vi "生成报告.vi"(0 "打印?":bool, 2 "输出簇":T1) -> ()   [LabVIEW 2010]
uses:
  <vilib>/Utility/NIReport.llb/NI_report.lvclass
  <vilib>/Utility/NIReport.llb/Append Report Text (str wrap).vi
  <vilib>/addons/_office/word.llb/Word Easy Table (str).vi
  <vilib>/addons/_office/NI_ReportGenerationToolkit.lvlib
panel:
  in  "序号":i32
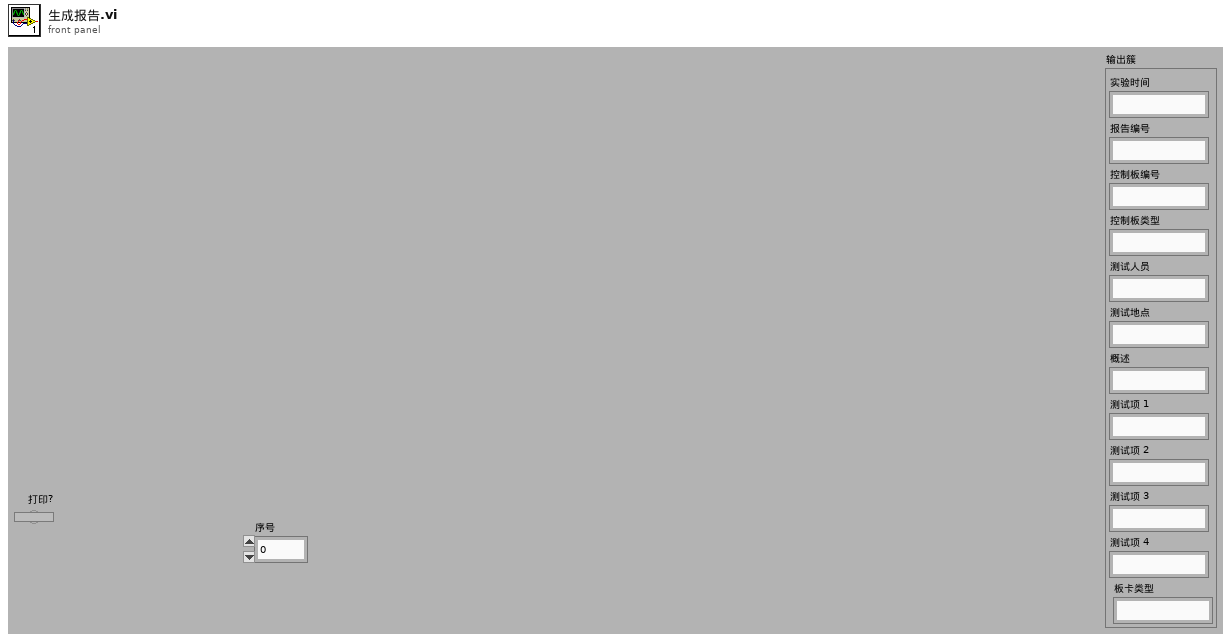
[diagram p1: front panel]
types:
  T1 = cluster{"实验时间":string, "报告编号":string, "控制板编号":string, "控制板类型":string, "测试人员":string, "测试地点":string, "概述":string, "测试项 1":string, "测试项 2":string, "测试项 3":string, "测试项 4":string, "板卡类型":string}
  T2 = cluster{"position (Excel)":cluster{"row":i32, "column":i32}, "name (Excel)":string, "bookmark (Word)":string}
  T3 = enum16{"maximized", "minimized", "normal", "no change"}
  T4 = enum16{"Standard Report", "HTML", "Word", "Excel"}
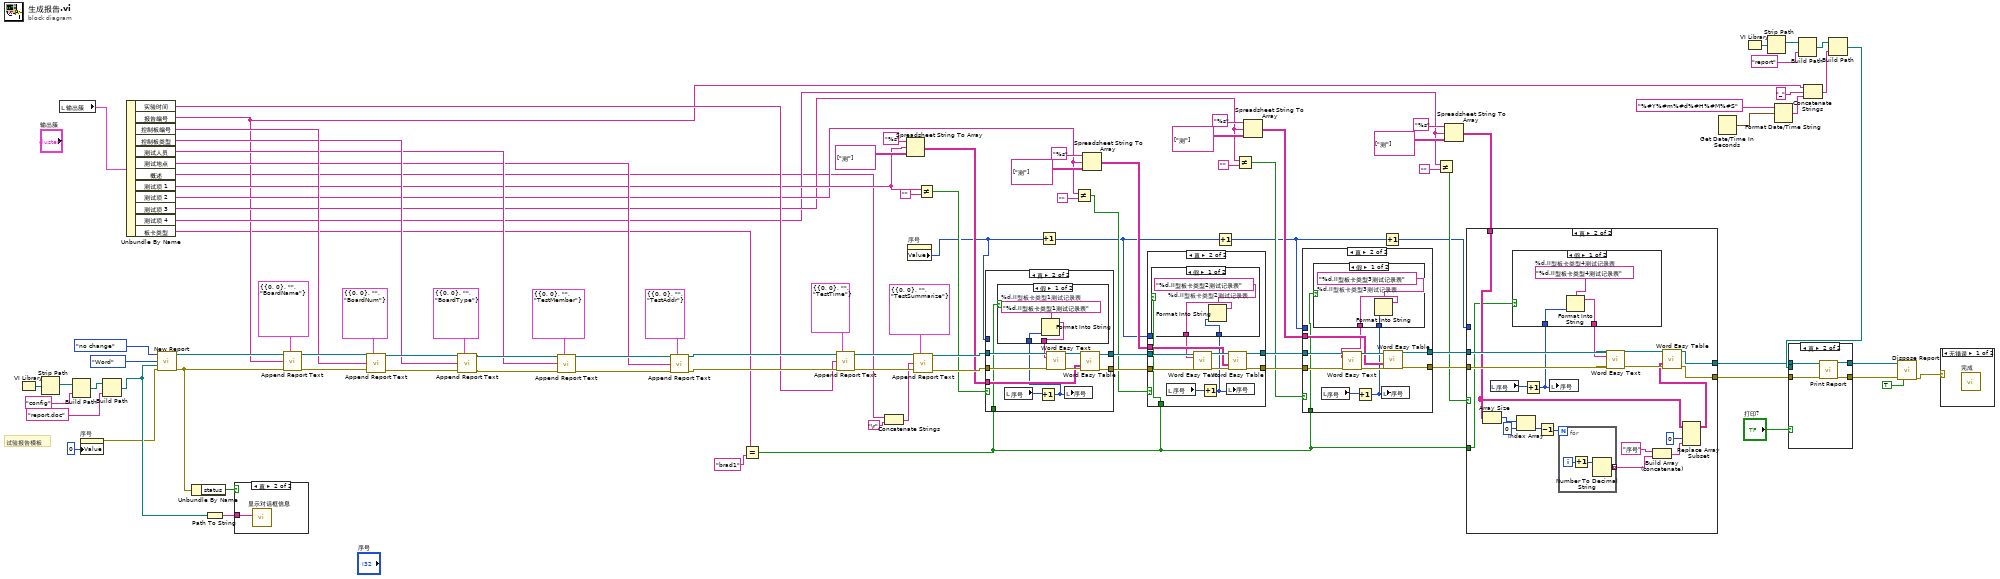
[diagram p0: block diagram]
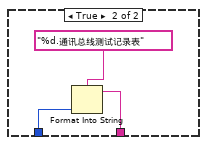
[diagram p3: hidden frame]
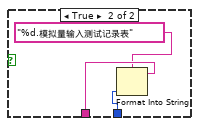
[diagram p5: hidden frame]
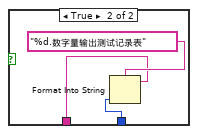
[diagram p7: hidden frame]
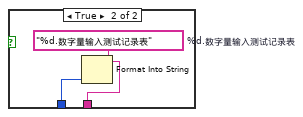
[diagram p9: hidden frame]
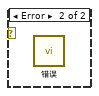
[diagram p10: hidden frame]
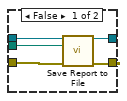
[diagram p11: hidden frame]
diagram:
  # "试验报告模板"
  n1 = VI Library() -> (path=w93:path)
  n2 = Strip Path(path=w93) -> (stripped path=w90:path)  [unwired: 1 out]
  n3 = local read "输出簇"() -> (w99:T1)
  n4 = Build Path(base path=w90, name or relative path="config") -> (appended path=w92:path)
  n5 = property on="序号" class="DigNum (严格)"("Value"=0 ("序号")) -> (error out=w44:errorcluster)  [unwired: 2 in, 1 out]
  n6 = Build Path(base path=w92, name or relative path="report.doc") -> (appended path=w96:path)
  n7 = Unbundle By Name(w99) -> ("实验时间"=w36:string, "报告编号"=w11:string, "控制板编号"=w40:string, "控制板类型"=w39:string, "测试人员"=w38:string, "测试地点"=w37:string, "概述"=w10:string, "测试项 1"=w31:string, "测试项 2"=w26:string, "测试项 3"=w20:string, "测试项 4"=w14:string, "板卡类型"=w2:string)
  n8 = call <vilib>:"New Report.vi"("window state (normal)"=T3."no change", "report type"=T4."Word", "template (empty)"=w96, "error in (no error)"=w44) -> ("report out"=w87:refnum<class "NI_report.lvclass">, "error out"=w86:errorcluster)  [unwired: 10 in]
  n9 = Unbundle By Name(w86) -> ("status"=w98:bool)
  n10 = Path To String(path=w96) -> (string=w97:string)
  n11 = case shown="真" w98 {
    tunnel: w97 -> [_ w100]
    frame False {
    }
    frame True {
      n12 = call "显示对话框信息"("Message"=w100) -> ()  [unwired: 9 in, 2 out]
    }
  }
  n13 = call-poly <vilib>:"Append Report Text.vi"("report in"=w87, "MS Office parameters"=T2 {"position (Excel)"={"row"=0, "column"=0}, "name (Excel)"="", "bookmark (Word)"="BoardName"}, "text"=w11, "error in (no error)"=w86) -> ("report out"=w72:refnum<class "NI_report.lvclass">, "error out"=w71:errorcluster)  [unwired: 8 in, 2 out]
  n14 = call-poly <vilib>:"Append Report Text.vi"("report in"=w72, "MS Office parameters"=T2 {"position (Excel)"={"row"=0, "column"=0}, "name (Excel)"="", "bookmark (Word)"="BoardNum"}, "text"=w40, "error in (no error)"=w71) -> ("report out"=w82:refnum<class "NI_report.lvclass">, "error out"=w81:errorcluster)  [unwired: 8 in, 2 out]
  n15 = call-poly <vilib>:"Append Report Text.vi"("report in"=w82, "MS Office parameters"=T2 {"position (Excel)"={"row"=0, "column"=0}, "name (Excel)"="", "bookmark (Word)"="BoardType"}, "text"=w39, "error in (no error)"=w81) -> ("report out"=w79:refnum<class "NI_report.lvclass">, "error out"=w78:errorcluster)  [unwired: 8 in, 2 out]
  n16 = call-poly <vilib>:"Append Report Text.vi"("report in"=w79, "MS Office parameters"=T2 {"position (Excel)"={"row"=0, "column"=0}, "name (Excel)"="", "bookmark (Word)"="TestMember"}, "text"=w38, "error in (no error)"=w78) -> ("report out"=w76:refnum<class "NI_report.lvclass">, "error out"=w75:errorcluster)  [unwired: 8 in, 2 out]
  n17 = call-poly <vilib>:"Append Report Text.vi"("report in"=w76, "MS Office parameters"=T2 {"position (Excel)"={"row"=0, "column"=0}, "name (Excel)"="", "bookmark (Word)"="TestAddr"}, "text"=w37, "error in (no error)"=w75) -> ("report out"=w74:refnum<class "NI_report.lvclass">, "error out"=w73:errorcluster)  [unwired: 8 in, 2 out]
  n18 = Equal?(x=w2, y="brad1") -> (x = y?=w1:bool)
  n19 = call-poly <vilib>:"Append Report Text.vi"("report in"=w74, "MS Office parameters"=T2 {"position (Excel)"={"row"=0, "column"=0}, "name (Excel)"="", "bookmark (Word)"="TestTime"}, "text"=w36, "error in (no error)"=w73) -> ("report out"=w49:refnum<class "NI_report.lvclass">, "error out"=w48:errorcluster)  [unwired: 8 in, 2 out]
  n20 = Concatenate Strings(w10, "\r") -> (w8:string)
  n21 = Spreadsheet String To Array(format string="%s" ("格式字符串"), spreadsheet string=w31, array type (2D Dbl)=string[][] [["测"]] ("数组类型(2D String)")) -> (array=w30:string[][])  [unwired: 1 in]
  n22 = property on="序号" class="DigNum (严格)"() -> ("Value"=w7:i32)  [unwired: 2 in, 2 out]
  n23 = call-poly <vilib>:"Append Report Text.vi"("report in"=w49, "MS Office parameters"=T2 {"position (Excel)"={"row"=0, "column"=0}, "name (Excel)"="", "bookmark (Word)"="TestSummarize"}, "text"=w8, "error in (no error)"=w48) -> ("report out"=w47:refnum<class "NI_report.lvclass">, "error out"=w46:errorcluster)  [unwired: 8 in, 2 out]
  n24 = Not Equal?(x=w31, y="") -> (x != y?=w34:bool)
  n25 = case shown="真" w34 {
    tunnel: [w102 w112] -> w56
    tunnel: [w101 w111] -> w54
    tunnel: w47 -> [w102 w109]
    tunnel: w46 -> [w101 w108]
    tunnel: w7 -> [_ _]
    tunnel: w30 -> [_ w107]
    tunnel: w1 -> [_ w105]
    frame False {
    }
    frame True {
      n26 = local read "序号"() -> (w104:i32)
      n27 = Increment(x=w104) -> (x+1=w103:i32)
      n28 = case shown="假" w105 {
        tunnel: [w115 w117] -> w106
        tunnel: w103 -> [w114 w119]
        frame False {
          w116 = "%d.II型板卡类型1测试记录表"  # %d.II型板卡类型1测试记录表
          n29 = Format Into String(format string=w116, w114) -> (resulting string=w115:string)  [unwired: 2 in, 1 out]
        }
        frame True {
          w118 = "%d.数字量输入测试记录表"  # %d.数字量输入测试记录表
          n30 = Format Into String(format string=w118, w119) -> (resulting string=w117:string)  [unwired: 2 in, 1 out]
        }
      }
      n31 = call <vilib>:"Word Easy Text.vi"("report in"=w109, "text"=w106, "error in (no error)"=w108) -> ("report out"=w113:refnum<class "NI_report.lvclass">, "error out"=w110:errorcluster)  [unwired: 10 in, 1 out]
      n32 = local write "序号"(w103) -> ()
      n33 = call-poly <vilib>:"Word Easy Table.vi"("report in"=w113, "data"=w107, "error in (no error)"=w110) -> ("report out"=w112:refnum<class "NI_report.lvclass">, "error out"=w111:errorcluster)  [unwired: 10 in, 1 out]
    }
  }
  n34 = Increment(x=w7) -> (x+1=w6:i32)
  n35 = Not Equal?(x=w26, y="") -> (x != y?=w25:bool)
  n36 = Spreadsheet String To Array(format string="%s" ("格式字符串"), spreadsheet string=w26, array type (2D Dbl)=string[][] [["测"]] ("数组类型(2D String)")) -> (array=w24:string[][])  [unwired: 1 in]
  n37 = case shown="真" w25 {
    tunnel: w56 -> [w121 w132]
    tunnel: [w121 w130] -> w55
    tunnel: w54 -> [w120 w129]
    tunnel: [w120 w127] -> w53
    tunnel: w6 -> [_ _]
    tunnel: w24 -> [_ w126]
    tunnel: w1 -> [_ w124]
    frame False {
    }
    frame True {
      n38 = local read "序号"() -> (w123:i32)
      n39 = Increment(x=w123) -> (x+1=w122:i32)
      n40 = case shown="假" w124 {
        tunnel: [w134 w136] -> w125
        tunnel: w122 -> [w135 w138]
        frame False {
          w133 = "%d.II型板卡类型2测试记录表"  # %d.II型板卡类型2测试记录表
          n41 = Format Into String(format string=w133, w135) -> (resulting string=w134:string)  [unwired: 2 in, 1 out]
        }
        frame True {
          n42 = Format Into String(format string="%d.数字量输出测试记录表", w138) -> (resulting string=w136:string)  [unwired: 2 in, 1 out]
        }
      }
      n43 = call <vilib>:"Word Easy Text.vi"("report in"=w132, "text"=w125, "error in (no error)"=w129) -> ("report out"=w131:refnum<class "NI_report.lvclass">, "error out"=w128:errorcluster)  [unwired: 10 in, 1 out]
      n44 = local write "序号"(w122) -> ()
      n45 = call-poly <vilib>:"Word Easy Table.vi"("report in"=w131, "data"=w126, "error in (no error)"=w128) -> ("report out"=w130:refnum<class "NI_report.lvclass">, "error out"=w127:errorcluster)  [unwired: 10 in, 1 out]
    }
  }
  n46 = Increment(x=w6) -> (x+1=w5:i32)
  n47 = Not Equal?(x=w20, y="") -> (x != y?=w19:bool)
  n48 = Spreadsheet String To Array(format string="%s" ("格式字符串"), spreadsheet string=w20, array type (2D Dbl)=string[][] [["测"]] ("数组类型(2D String)")) -> (array=w18:string[][])  [unwired: 1 in]
  n49 = case shown="真" w19 {
    tunnel: w55 -> [w140 w151]
    tunnel: w53 -> [w139 w149]
    tunnel: [w140 w147] -> w52
    tunnel: [w139 w146] -> w51
    tunnel: w5 -> [_ _]
    tunnel: w18 -> [_ w145]
    tunnel: w1 -> [_ w143]
    frame False {
    }
    frame True {
      n50 = local read "序号"() -> (w142:i32)
      n51 = Increment(x=w142) -> (x+1=w141:i32)
      n52 = case shown="假" w143 {
        tunnel: [w153 w156] -> w144
        tunnel: w141 -> [w154 w157]
        frame False {
          w152 = "%d.II型板卡类型3测试记录表"  # %d.II型板卡类型3测试记录表
          n53 = Format Into String(format string=w152, w154) -> (resulting string=w153:string)  [unwired: 2 in, 1 out]
        }
        frame True {
          n54 = Format Into String(format string="%d.模拟量输入测试记录表", w157) -> (resulting string=w156:string)  [unwired: 2 in, 1 out]
        }
      }
      n55 = call <vilib>:"Word Easy Text.vi"("report in"=w151, "text"=w144, "error in (no error)"=w149) -> ("report out"=w150:refnum<class "NI_report.lvclass">, "error out"=w148:errorcluster)  [unwired: 10 in, 1 out]
      n56 = local write "序号"(w141) -> ()
      n57 = call-poly <vilib>:"Word Easy Table.vi"("report in"=w150, "data"=w145, "error in (no error)"=w148) -> ("report out"=w147:refnum<class "NI_report.lvclass">, "error out"=w146:errorcluster)  [unwired: 10 in, 1 out]
    }
  }
  n58 = Increment(x=w5) -> (x+1=w4:i32)
  n59 = Not Equal?(x=w14, y="") -> (x != y?=w13:bool)
  n60 = Spreadsheet String To Array(format string="%s" ("格式字符串"), spreadsheet string=w14, array type (2D Dbl)=string[][] [["测"]] ("数组类型(2D String)")) -> (array=w12:string[][])  [unwired: 1 in]
  n61 = case shown="真" w13 {
    tunnel: [w159 w179] -> w58
    tunnel: [w158 w178] -> w57
    tunnel: w52 -> [w159 w177]
    tunnel: w51 -> [w158 w176]
    tunnel: w4 -> [_ _]
    tunnel: w12 -> [_ w164]
    tunnel: w1 -> [_ w162]
    frame False {
    }
    frame True {
      n62 = Array Size(array=w164) -> (size(s)=w165:i32[])
      n63 = local read "序号"() -> (w161:i32)
      n64 = Index Array(array=w165, index=0 ("索引")) -> (element=w168:i32)
      n65 = Increment(x=w161) -> (x+1=w160:i32)
      n66 = case shown="假" w162 {
        tunnel: [w182 w185] -> w173
        tunnel: w160 -> [w180 w183]
        frame False {
          w181 = "%d.II型板卡类型4测试记录表"  # %d.II型板卡类型4测试记录表
          n67 = Format Into String(format string=w181, w180) -> (resulting string=w182:string)  [unwired: 2 in, 1 out]
        }
        frame True {
          n68 = Format Into String(format string="%d.通讯总线测试记录表", w183) -> (resulting string=w185:string)  [unwired: 2 in, 1 out]
        }
      }
      n69 = Decrement(x=w168) -> (x-1=w169:i32)
      n70 = local write "序号"(w160) -> ()
      n71 = for {
        N: w169 -> [_]
        tunnel: [w186] -> w171 mode=indexing
        i -> [w188]
        n72 = Increment(x=w188) -> (x+1=w187:i32)
        n73 = Number To Decimal String(number=w187) -> (decimal integer string=w186:string)  [unwired: 1 in]
      }
      n74 = call <vilib>:"Word Easy Text.vi"("report in"=w177, "text"=w173, "error in (no error)"=w176) -> ("report out"=w175:refnum<class "NI_report.lvclass">, "error out"=w174:errorcluster)  [unwired: 10 in, 1 out]
      n75 = Build Array (concatenate)("序号", w171) -> (w172:string[])
      n76 = Replace Array Subset(array=w164, new element=w172, index (col)=0 ("索引 (行)")) -> (w163:string[][])  [unwired: 1 in]
      n77 = call-poly <vilib>:"Word Easy Table.vi"("report in"=w175, "data"=w163, "error in (no error)"=w174) -> ("report out"=w179:refnum<class "NI_report.lvclass">, "error out"=w178:errorcluster)  [unwired: 10 in, 1 out]
    }
  }
  n78 = Get Date/Time In Seconds() -> (seconds since 1Jan1904=w65:timestamp)
  n79 = VI Library() -> (path=w66:path)
  n80 = Strip Path(path=w66) -> (stripped path=w69:path)  [unwired: 1 out]
  n81 = Format Date/Time String(time format string (%c)="%#Y%#m%#d%#H%#M%#S" ("时间格式字符串(%c)"), seconds (now)=w65) -> (date/time string=w43:string)  [unwired: 1 in]
  n82 = Build Path(base path=w69, name or relative path="report") -> (appended path=w67:path)
  n83 = Concatenate Strings(w11, "_", w43) -> (w41:string)
  n84 = Build Path(base path=w67, name or relative path=w41) -> (appended path=w60:path)
  n85 = case shown="真" "打印?" {
    tunnel: w58 -> [w193 w197]
    tunnel: w57 -> [w192 w196]
    tunnel: [w191 w195] -> w63
    tunnel: [w190 w194] -> w62
    tunnel: w60 -> [w189 _]
    frame False {
      n86 = call-dynamic "Save Report to File.vi"("report in"=w193, "report file path"=w189, "error in (no error)"=w192) -> ("report out"=w191:refnum<class "NI_report.lvclass">, "error out"=w190:errorcluster)  [unwired: 11 in]
    }
    frame True {
      n87 = call-dynamic "Print Report.vi"("report in"=w197, "error in (no error)"=w196) -> ("report out"=w195:refnum<class "NI_report.lvclass">, "error out"=w194:errorcluster)  [unwired: 12 in]
    }
  }
  n88 = call-dynamic "Dispose Report.vi"("report in"=w63, "error in (no error)"=w62, "close report? (T)"=TRUE) -> ("error out"=w59:errorcluster)  [unwired: 12 in]
  n89 = case shown="无错误" w59 {
    frame No Error {
      n90 = call "完成"() -> ()  [unwired: 10 in, 2 out]
    }
    frame Error {
      n91 = call "错误"() -> ()  [unwired: 10 in, 2 out]
    }
  }
